vi "Create Character.vi"() -> (3 "Normal Game":T1)   [LabVIEW 2018]
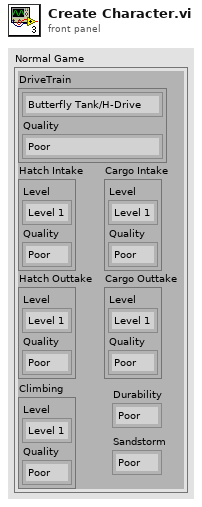
[diagram p1: front panel]
types:
  T1 = cluster{"DriveTrain":cluster{enum16{"Butterfly Tank/H-Drive", "Butterfly-Tank/Tank", "Tread", "Strafe", "Swerve", "Tank Traction"}, "Quality":enum16{"Poor", "Good", "Excellent"}}, "Cargo Intake":cluster{"Level":enum16{"Level 1", "Level 2", "Level 3"}, "Quality":enum16{"Poor", "Good", "Excellent"}}, "Hatch Intake":cluster{"Level":enum16{"Level 1", "Level 2", "Level 3"}, "Quality":enum16{"Poor", "Good", "Excellent"}}, "Cargo Outtake":cluster{"Level":enum16{"Level 1", "Level 2", "Level 3"}, "Quality":enum16{"Poor", "Good", "Excellent"}}, "Hatch Outtake":cluster{"Level":enum16{"Level 1", "Level 2", "Level 3"}, "Quality":enum16{"Poor", "Good", "Excellent"}}, "Climbing":cluster{"Level":enum16{"Level 1", "Level 2", "Level 3"}, "Quality":enum16{"Poor", "Good", "Excellent"}}, "Durability":enum16{"Poor", "Good", "Excellent"}, "Sandstorm":enum16{"Poor", "Good", "Excellent"}}
  T2 = cluster{enum16{"Butterfly Tank/H-Drive", "Butterfly-Tank/Tank", "Tread", "Strafe", "Swerve", "Tank Traction"}, "Quality":enum16{"Poor", "Good", "Excellent"}}
  T3 = enum16{"Butterfly Tank/H-Drive", "Butterfly-Tank/Tank", "Tread", "Strafe", "Swerve", "Tank Traction"}
  T4 = cluster{"Level":enum16{"Level 1", "Level 2", "Level 3"}, "Quality":enum16{"Poor", "Good", "Excellent"}}
  T5 = cluster{"DriveTrain":cluster{enum16{"Butterfly Tank/H-Drive", "Butterfly-Tank/Tank", "Tread", "Strafe", "Swerve", "Tank Traction"}, "Quality":enum16{"Poor", "Good", "Excellent"}}, "Cargo Intake":cluster{"Level":enum16{"Level 1", "Level 2", "Level 3"}, "Quality":enum16{"Poor", "Good", "Excellent"}}, "Hatch Intake":cluster{"Level":enum16{"Level 1", "Level 2", "Level 3"}, "Quality":enum16{"Poor", "Good", "Excellent"}}, "Cargo Outtake":cluster{"Level":enum16{"Level 1", "Level 2", "Level 3"}, "Quality":enum16{"Poor", "Good", "Excellent"}}, "Hatch Outtake":cluster{"Level":enum16{"Level 1", "Level 2", "Level 3"}, "Quality":enum16{"Poor", "Good", "Excellent"}}, "Climbing":cluster{"Level":enum16{"Level 1", "Level 2", "Level 3"}, "Quality":enum16{"Poor", "Good", "Excellent"}}, "Quality":enum16{"Poor", "Good", "Excellent"}, "Quality":enum16{"Poor", "Good", "Excellent"}}
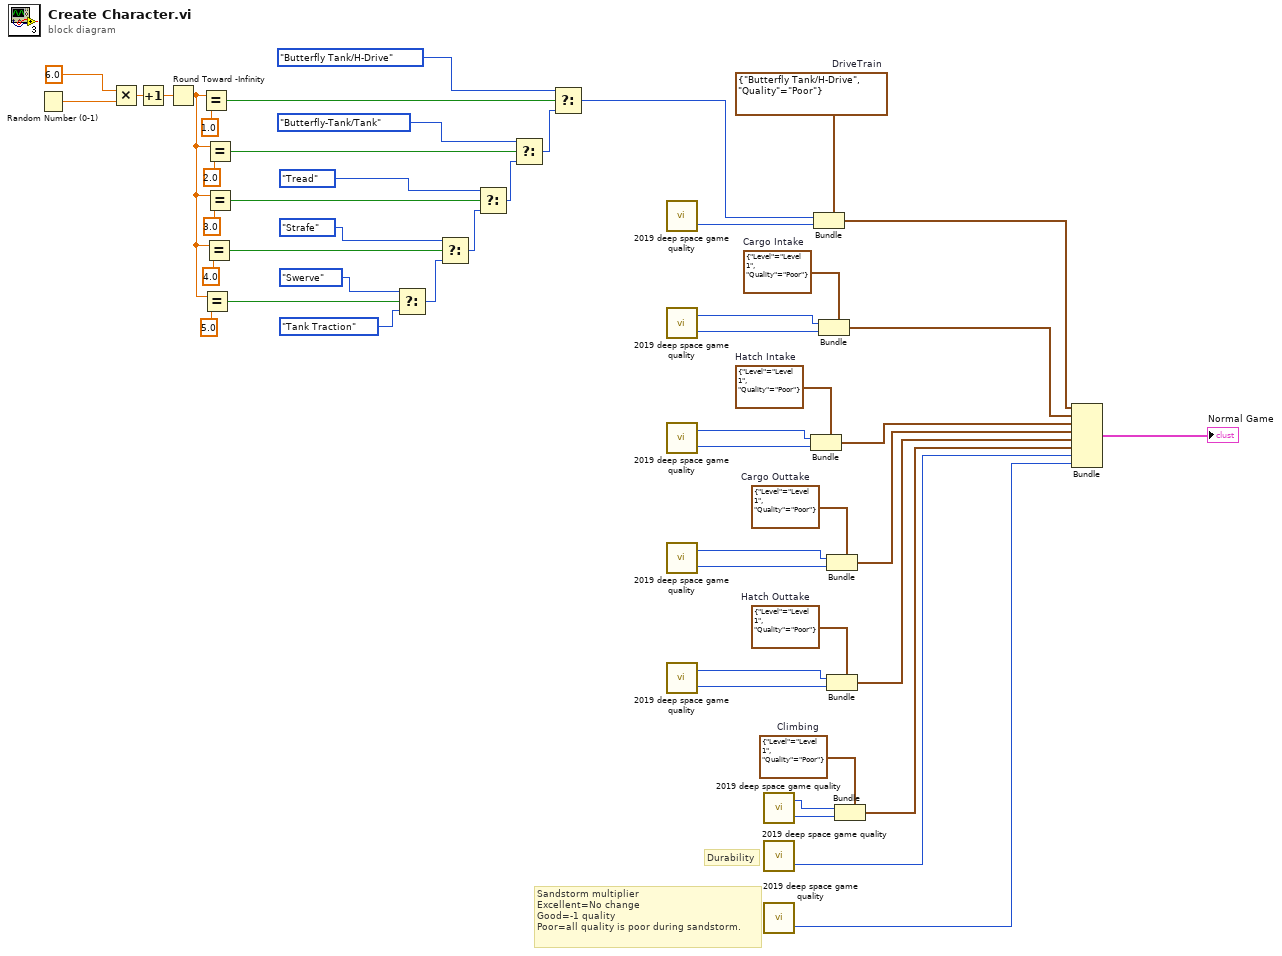
[diagram p0: block diagram]
diagram:
  w44 = T2 {enum."Butterfly Tank/H-Drive", "Quality"=enum."Poor"}  # DriveTrain
  w18 = T4 {"Level"=enum."Level 1", "Quality"=enum."Poor"}  # Climbing
  w17 = T4 {"Level"=enum."Level 1", "Quality"=enum."Poor"}  # Hatch Outtake
  w16 = T4 {"Level"=enum."Level 1", "Quality"=enum."Poor"}  # Cargo Outtake
  w15 = T4 {"Level"=enum."Level 1", "Quality"=enum."Poor"}  # Hatch Intake
  w14 = T4 {"Level"=enum."Level 1", "Quality"=enum."Poor"}  # Cargo Intake
  # "Durability"
  # "Sandstorm multiplier\nExcellent=No change\nGood=-1 quality\nPoor=all quality is poor during sandstorm."
  n1 = Random Number (0-1)() -> (number: 0 to 1=w26:dbl)
  n2 = Multiply(x=6.0, y=w26) -> (x*y=w24:dbl)
  n3 = Increment(x=w24) -> (x+1=w23:dbl)
  n4 = Round Toward -Infinity(1:w23) -> (0:w51:dbl)
  n5 = Equal?(x=w51, y=1.0) -> (x = y?=w21:bool)
  n6 = Equal?(x=w51, y=5.0) -> (x = y?=w39:bool)
  n7 = Equal?(x=w51, y=4.0) -> (x = y?=w38:bool)
  n8 = Equal?(x=w51, y=2.0) -> (x = y?=w33:bool)
  n9 = Equal?(x=w51, y=3.0) -> (x = y?=w35:bool)
  n10 = Select(t=T3."Swerve", s=w39, f=T3."Tank Traction") -> (s? t:f=w30:T3)
  n11 = Select(t=T3."Strafe", s=w38, f=w30) -> (s? t:f=w29:T3)
  n12 = Select(t=T3."Tread", s=w35, f=w29) -> (s? t:f=w28:T3)
  n13 = Select(t=T3."Butterfly-Tank/Tank", s=w33, f=w28) -> (s? t:f=w19:T3)
  n14 = Select(t=T3."Butterfly Tank/H-Drive", s=w21, f=w19) -> (s? t:f=w43:T3)
  n15 = call "2019 deep space game quality.vi"() -> ("Quality"=w13:enum16{"Poor", "Good", "Excellent"})  [unwired: 4 in, 1 out]
  n16 = call "2019 deep space game quality.vi"() -> ("Quality"=w12:enum16{"Poor", "Good", "Excellent"}, "Level"=w11:enum16{"Level 1", "Level 2", "Level 3"})  [unwired: 4 in]
  n17 = call "2019 deep space game quality.vi"() -> ("Quality"=w9:enum16{"Poor", "Good", "Excellent"}, "Level"=w10:enum16{"Level 1", "Level 2", "Level 3"})  [unwired: 4 in]
  n18 = call "2019 deep space game quality.vi"() -> ("Quality"=w7:enum16{"Poor", "Good", "Excellent"}, "Level"=w8:enum16{"Level 1", "Level 2", "Level 3"})  [unwired: 4 in]
  n19 = call "2019 deep space game quality.vi"() -> ("Quality"=w5:enum16{"Poor", "Good", "Excellent"}, "Level"=w6:enum16{"Level 1", "Level 2", "Level 3"})  [unwired: 4 in]
  n20 = call "2019 deep space game quality.vi"() -> ("Quality"=w3:enum16{"Poor", "Good", "Excellent"}, "Level"=w4:enum16{"Level 1", "Level 2", "Level 3"})  [unwired: 4 in]
  n21 = call "2019 deep space game quality.vi"() -> ("Quality"=w2:enum16{"Poor", "Good", "Excellent"})  [unwired: 4 in, 1 out]
  n22 = call "2019 deep space game quality.vi"() -> ("Quality"=w1:enum16{"Poor", "Good", "Excellent"})  [unwired: 4 in, 1 out]
  n23 = Bundle(cluster=w15, "Level"=w10, "Quality"=w9) -> (w47:T4)
  n24 = Bundle(cluster=w44, w43, "Quality"=w13) -> (w45:T2)
  n25 = Bundle(cluster=w14, "Level"=w11, "Quality"=w12) -> (w46:T4)
  n26 = Bundle(cluster=w16, "Level"=w8, "Quality"=w7) -> (w48:T4)
  n27 = Bundle(cluster=w17, "Level"=w6, "Quality"=w5) -> (w49:T4)
  n28 = Bundle(cluster=w18, "Level"=w4, "Quality"=w3) -> (w50:T4)
  n29 = Bundle("DriveTrain"=w45, "Cargo Intake"=w46, "Hatch Intake"=w47, "Cargo Outtake"=w48, "Hatch Outtake"=w49, "Climbing"=w50, "Quality"=w2, "Quality"=w1) -> (→"Normal Game":T5)  [unwired: 1 in]
